vi "Get niScope_ReadResult.vi"(8 "error in (no error)":errorcluster, 11 "gRPCid":T3) -> (0 "error out":errorcluster, 2 "Message Data":T1, 3 "gRPCid out":T3)   [LabVIEW 2019, in "TestServer.lvlib" / "TestServer.lvclass"]
uses:
  TestServer.lvclass
  gRPC lvSupport/Server API/typeDefs/grpcId.ctl
  niScope_ReadResult_Data.ctl
  niScope_ScopeWaveformInfo/niScope_ScopeWaveformInfo_Data.ctl
  a51dd2a7-b5c1-4c09-9df4-8cd9d3bd0c19.vi
  gRPC lvSupport/Server API/Server/Get Server DLL Path.vi
  gRPC lvSupport/gprc-lvsupport.lvlib
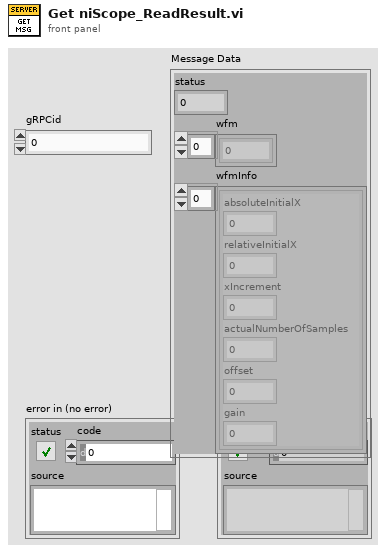
[diagram p1: front panel]
types:
  T1 = typedef "TestServer.lvlib/TestServer.lvclass/niScope_ReadResult_Data.ctl" = cluster{"status":i32, "wfm":dbl[], "wfmInfo":T2[]}
  T2 = typedef "TestServer.lvlib/TestServer.lvclass/niScope_ScopeWaveformInfo_Data.ctl" = cluster{"absoluteInitialX":dbl, "relativeInitialX":dbl, "xIncrement":dbl, "actualNumberOfSamples":i32, "offset":dbl, "gain":dbl}
  T3 = typedef "TestServer.lvlib/gprc-lvsupport.lvlib/grpcId.ctl" = u64
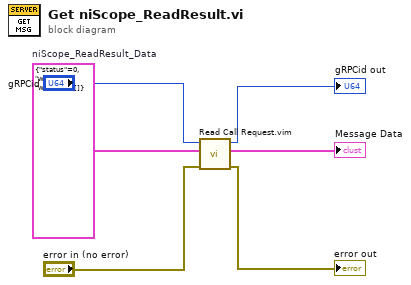
[diagram p0: block diagram]
diagram:
  w2 = T1 {"status"=0, "wfm"=[], "wfmInfo"=[]}  # niScope_ReadResult_Data
  n1 = call "Read Call Request.vim"("error in (no error)"="error in (no error)", "Data Type"=w2, "gRPCid in"="gRPCid") -> ("error out"=→"error out":errorcluster, "Request Data"=→"Message Data":T1, "gRPCid out"=→"gRPCid out":T3)  [unwired: 6 in]
